vi "test Create and Look Into Rx Execution Unit Map_RandomLabelsPerChannel.vi"(8 "error in":errorcluster, 11 "TestCase in":refnum<class "Engine.lvclass">) -> (0 "error out":errorcluster, 3 "TestCase out":refnum<class "Engine.lvclass">)   [LabVIEW 2020, in "Engine.lvclass"]
uses:
  Engine.lvclass
  Shared/Parameter Definition.ctl
  Encoding and Decoding/Encoding.ctl
  Shared/RT Hardware Channel Settings.ctl
  Shared/RT Label Settings.ctl
  Shared/Label.ctl
  Shared/RT Parameters.ctl
  <vilib>/NI VeriStand/Custom Device API/Custom Device Item Ref.ctl
  Shared/Transfer Type.ctl
  <vilib>/NI VeriStand/Custom Device API/Data Reference.ctl
  <vilib>/numeric/Random Number (Range) U64.vi
  <vilib>/numeric/sub_Random U32.vi
  <vilib>/addons/_JKI Toolkits/VI Tester/TestCase.llb/TestCase.lvclass
  Engine/Custom Device/Custom Device.lvlib
  <vilib>/NI VeriStand/Custom Device API/Custom Device API.lvlib
  Encoding and Decoding/Encoding and Decoding.lvlib
  C:/Program Files (x86)/National Instruments/LabVIEW 2020/vi.lib/addons/_JKI Toolkits/VI Tester/TestCase.llb/TestCase.lvclass
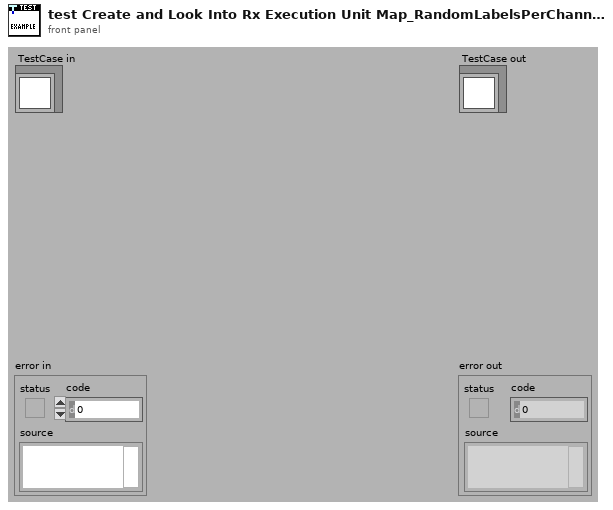
[diagram p1: front panel]
types:
  T1 = typedef "Parameter Definition.ctl" = cluster{"start index":i32, "size":i32, "encoding":T2, "signed":bool, "scale multiplier":dbl, "scale offset":dbl}
  T2 = typedef "Encoding and Decoding.lvlib/Encoding.ctl" = enum16{"BNR", "BCD", "Discrete"}
  T3 = typedef "RT Hardware Channel Settings.ctl" = cluster{"channel #":u16, "channel handle":u64, "labels settings for RT":T4[]}
  T4 = typedef "RT Label Settings.ctl" = cluster{"Name":string, "xmlName":string, "label":T5, "transfer period":u32, "SDI_Enabled":bool, "SDI":u8, "parameter driver data":T6, "transfer type":T8, "has timestamp?":bool, "Label Disable/Trigger Channel Reference":T7, "Message Handle":u64, "Initialized?":bool, "Word Initial Raw Value":u32, "Label Timestamp Channel Data Reference":T9, "disabled":bool}
  T5 = typedef "Label.ctl" = u8
  T6 = typedef "RT Parameters.ctl" = cluster{"parameter definitions":T1[], "Rx values":dbl[], "Tx parameter refs":T7[]}
  T7 = typedef "Custom Device API.lvlib/Custom Device Item Ref.ctl" = u64
  T8 = typedef "Transfer Type.ctl" = enum16{"Scheduled", "Acyclic", "Block", "Strobe"}
  T9 = typedef "Custom Device API.lvlib/Data Reference.ctl" = i32
  T10 = cluster{"channel index":i32, "label index":i32, "start index":i32, "parameters":i32, "timestamp index":i32}
  T11 = typedef "Map of Identifiers to Indexes.ctl" = map{cluster{"Port":u8, "Label":u8, "SDI":u8}, cluster{"channel index":i32, "label index":i32, "start index":i32, "parameters":i32, "timestamp index":i32}}
  T12 = cluster{"channel index":i32, "label index":i32, "start index":i32, "parameters":i32, "timestamp index":i32}[]
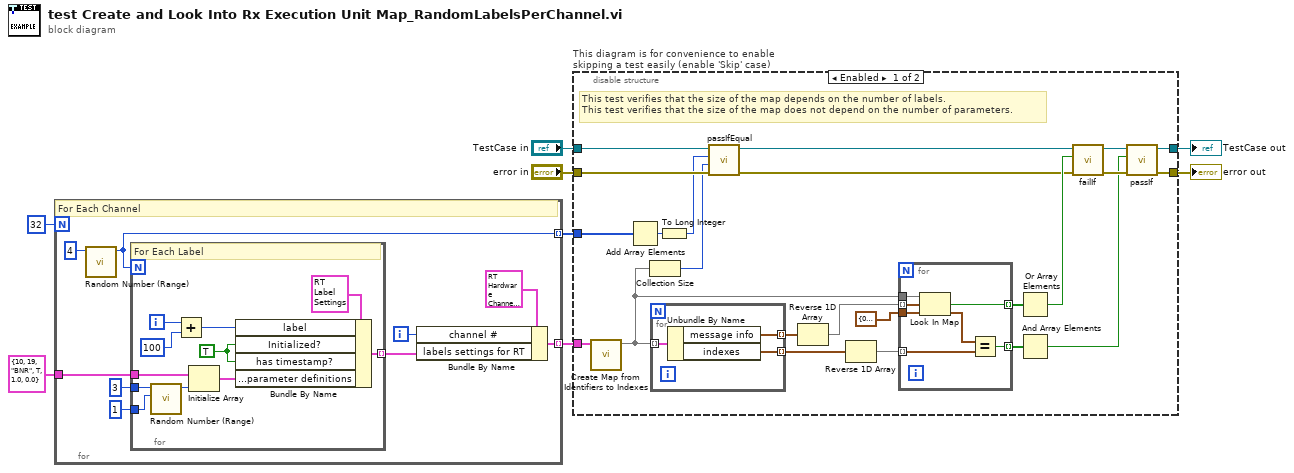
[diagram p0: block diagram]
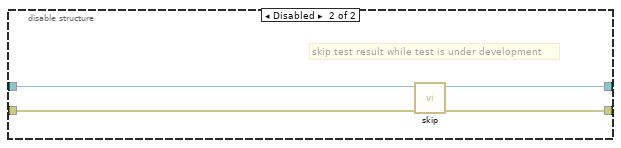
[diagram p2: hidden frame]
diagram:
  n1 = for {
    N: 32 -> [_]
    tunnel: T1 {"start index"=10, "size"=19, "encoding"=enum."BNR", "signed"=TRUE, "scale multiplier"=1.0, "scale offset"=0.0} ("parameter definition out") -> [w16]
    tunnel: [w12] -> w2 mode=indexing
    tunnel: [w11] -> w1 mode=indexing
    i -> [w13]
    # "For Each Channel"
    n2 = call-poly <vilib>:"Random Number (Range).vi"("upper bound (100)"=u64 4) -> ("number"=w11:u64)  [unwired: 10 in]
    n3 = for {
      N: w11 -> [_]
      tunnel: w16 -> [w24]
      tunnel: [w23] -> w15 mode=indexing
      tunnel: u64 3 ("upper bound (100)") -> [w19]
      tunnel: u64 1 ("upper bound (100)") -> [w18]
      i -> [w28]
      w21 = TRUE ("Initialized?")
      # "For Each Label"
      n4 = call-poly <vilib>:"Random Number (Range).vi"("lower bound (0)"=w18, "upper bound (100)"=w19) -> ("number"=w22:u64)  [unwired: 9 in]
      n5 = Add(x=w28, y=100) -> (x+y=w26:i32)
      n6 = Initialize Array(w24, w22) -> (w25:T1[])
      n7 = Bundle By Name(cluster=T4 {"Name"="", "xmlName"="", "label"=0, "transfer period"=0, "SDI_Enabled"=FALSE, "SDI"=0, "parameter driver data"={"parameter definitions"=[], "Rx values"=[], "Tx parameter refs"=[]}, "transfer type"=enum."Scheduled", "has timestamp?"=FALSE, "Label Disable/Trigger Channel Reference"=0, "Message Handle"=0, "Initialized?"=FALSE, "Word Initial Raw Value"=0, "Label Timestamp Channel Data Reference"=0, "disabled"=FALSE} ("label settings for RT"), "label"=w26, "Initialized?"=w21, "has timestamp?"=w21, "parameter driver data.parameter definitions"=w25) -> (w23:T4)
    }
    n8 = Bundle By Name(cluster=T3 {"channel #"=1, "channel handle"=0, "labels settings for RT"=[{"Name"="", "xmlName"="", "label"=11, "transfer period"=0, "SDI_Enabled"=FALSE, "SDI"=0, "parameter driver data"={"parameter definitions"=[{"start index"=10, "size"=16, "encoding"=enum."BCD", "signed"=TRUE, "scale multiplier"=1.0, "scale offset"=0.0}], "Rx values"=[], "Tx parameter refs"=[]}, "transfer type"=enum."Scheduled", "has timestamp?"=TRUE, "Label Disable/Trigger Channel Reference"=0, "Message Handle"=0, "Initialized?"=TRUE, "Word Initial Raw Value"=0, "Label Timestamp Channel Data Reference"=0, "disabled"=FALSE}, {"Name"="", "xmlName"="", "label"=55, "transfer period"=0, "SDI_Enabled"=FALSE, "SDI"=0, "parameter driver data"={"parameter definitions"=[{"start index"=15, "size"=11, "encoding"=enum."BNR", "signed"=FALSE, "scale multiplier"=0.0, "scale offset"=0.0}], "Rx values"=[], "Tx parameter refs"=[]}, "transfer type"=enum."Scheduled", "has timestamp?"=FALSE, "Label Disable/Trigger Channel Reference"=0, "Message Handle"=0, "Initialized?"=TRUE, "Word Initial Raw Value"=0, "Label Timestamp Channel Data Reference"=0, "disabled"=FALSE}, {"Name"="", "xmlName"="", "label"=77, "transfer period"=0, "SDI_Enabled"=FALSE, "SDI"=0, "parameter driver data"={"parameter definitions"=[{"start index"=10, "size"=4, "encoding"=enum."BCD", "signed"=FALSE, "scale multiplier"=0.0, "scale offset"=0.0}, {"start index"=14, "size"=2, "encoding"=enum."BNR", "signed"=FALSE, "scale multiplier"=0.0, "scale offset"=0.0}, {"start index"=16, "size"=12, "encoding"=enum."BNR", "signed"=FALSE, "scale multiplier"=0.0, "scale offset"=0.0}], "Rx values"=[], "Tx parameter refs"=[]}, "transfer type"=enum."Scheduled", "has timestamp?"=FALSE, "Label Disable/Trigger Channel Reference"=0, "Message Handle"=0, "Initialized?"=TRUE, "Word Initial Raw Value"=0, "Label Timestamp Channel Data Reference"=0, "disabled"=FALSE}]} ("RT hardware channel"), "channel #"=w13, "labels settings for RT"=w15) -> (w12:T3)
  }
  n9 = disable-structure "This diagram is for convenience to enable skipping a test easily (enable 'Skip' case)" shown="Enabled" {
    disable-tunnel: "TestCase in" -> [w34 w65]
    disable-tunnel: [w51 w63] -> w5
    disable-tunnel: [w50 w64] -> w7
    disable-tunnel: "error in" -> [w33 w62]
    disable-tunnel: w2 -> [w49 _]
    disable-tunnel: w1 -> [w30 _]
    frame Enabled {
      # "This test verifies that the size of the map depends on the number of labels.\nThis test verifies that the size of the map does not depend on the number of parameters."
      n10 = call "Create Map from Identifiers to Indexes.vi"("RT hardware channel data"=w49) -> ("map from identifiers to indexes"=w37:T11)  [unwired: 10 in]
      n11 = Add Array Elements(numeric array=w30) -> (sum=w31:u64)
      n12 = Collection Size(1:w37) -> (0:w32:i32)
      n13 = for {
        tunnel: w37 -> [w61] mode=indexing
        tunnel: [w60] -> w48 mode=indexing
        tunnel: [w59] -> w47 mode=indexing
        n14 = Unbundle By Name(w61) -> ("message info"=w60:cluster{"Port":u8, "Label":u8, "SDI":u8}, "indexes"=w59:T10)
      }
      n15 = To Long Integer(number=w31) -> (32bit integer=w29:i32)
      n16 = call-dynamic "passIfEqual.vi"("error in (no error)"=w33, "y"=w32, "x"=w29, "TestCase in"=w34) -> ("error out"=w35:errorcluster, "TestCase out"=w36:refnum<class "Engine.lvclass">)  [unwired: 6 in]
      n17 = Reverse 1D Array(array=w48) -> (reversed array=w46:cluster{"Port":u8, "Label":u8, "SDI":u8}[])
      n18 = Reverse 1D Array(array=w47) -> (reversed array=w40:T12)
      n19 = for {
        tunnel: w37 -> [w58]
        tunnel: w46 -> [w57] mode=indexing
        tunnel: T10 {"channel index"=0, "label index"=0, "start index"=0, "parameters"=0, "timestamp index"=0} ("default value") -> [w56]
        tunnel: [w55] -> w44 mode=indexing
        tunnel: w40 -> [w53] mode=indexing
        tunnel: [w52] -> w39 mode=indexing
        n20 = Look In Map(map=w58, key=w57, default value=w56) -> (key not found?=w55:bool, value=w54:T10)
        n21 = Equal?(x=w54, y=w53) -> (x = y?=w52:bool)
      }
      n22 = Or Array Elements(Boolean array=w44) -> (logical OR=w43:bool)
      n23 = And Array Elements(Boolean array=w39) -> (logical AND=w38:bool)
      n24 = call-dynamic "failIf.vi"("error in (no error)"=w35, "fail"=w43, "TestCase in"=w36) -> ("error out"=w41:errorcluster, "TestCase out"=w42:refnum<class "Engine.lvclass">)  [unwired: 7 in]
      n25 = call-dynamic "passIf.vi"("error in (no error)"=w41, "pass"=w38, "TestCase in"=w42) -> ("error out"=w50:errorcluster, "TestCase out"=w51:refnum<class "Engine.lvclass">)  [unwired: 7 in]
    }
    frame Disabled {
      # "skip test result while test is under development"
      n26 = call <vilib>:"skip.vi"("error in (no error)"=w62, "TestCase in"=w65) -> ("error out"=w64:errorcluster, "TestCase out"=w63:refnum<class "Engine.lvclass">)  [unwired: 8 in]
    }
  }
  "error out" <- w7
  "TestCase out" <- w5
